vi "OpenDeviceBySN.vi"(2 "error in (no error)":errorcluster, 3 "SN":string, 4 "IGxFactory":refnum<k24>) -> (0 "error out":errorcluster, 1 "IGxDevice":refnum<k24>)   [LabVIEW 2013, in "GxLVlib.lvlib"]
uses:
  GxLVlib.lvlib
  F:/GxILibrary/Labview/trunk/private/dev/src/C#/x86/GxLVLib/dll/GxIAPINET.dll
  private/dev/src/C#/x86/GxLVLib/dll/GxIAPINET.dll
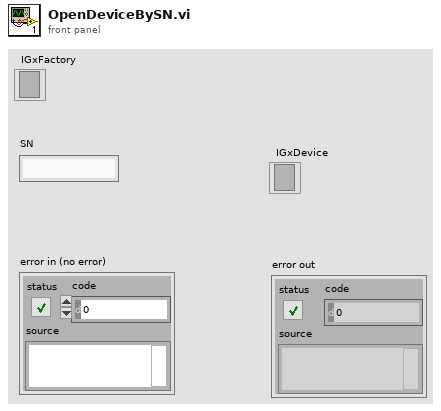
[diagram p1: front panel]
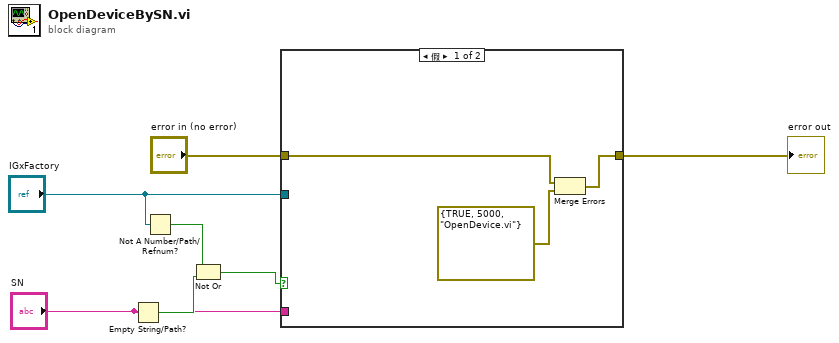
[diagram p0: block diagram]
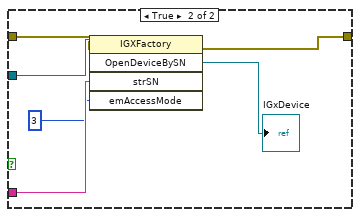
[diagram p2: hidden frame]
diagram:
  n1 = Empty String/Path?(string/path="SN") -> (empty?=w6:bool)
  n2 = Not A Number/Path/Refnum?(number/path/refnum="IGxFactory") -> (NaN/Path/Refnum?=w7:bool)
  n3 = Not Or(1:w6, 2:w7) -> (0:w5:bool)
  n4 = case shown="假" w5 {
    tunnel: "error in (no error)" -> [w10 w13]
    tunnel: [w8 w12] -> w3
    tunnel: "IGxFactory" -> [_ w16]
    tunnel: "SN" -> [_ w15]
    frame False {
      n5 = Merge Errors(w10, errorcluster {TRUE, 5000, "OpenDevice.vi"}) -> (w8:errorcluster)
    }
    frame True {
      n6 = invoke class="IGXFactory" method="OpenDeviceBySN"(reference=w16, error in=w13, "strSN"=w15, "emAccessMode"=3) -> (error out=w12:errorcluster, "OpenDeviceBySN"=→"IGxDevice":refnum<k24>)  [unwired: 1 in, 3 out]
    }
  }
  "error out" <- w3
